vi "Empty_Complete.vi"(11 "input cluster":T1={"system"={"info"={"menuSelect"=0, "version"=0, "serial"="Test Sample", "captureActive"=FALSE, "captureBegin"=FALSE, "emptyAndRefill"=FALSE}, "userInfo"={"operatorName"="", "date"=timestamp(2713993200 s since 1904-01-01)}, "camera"={"exposureTime"=0, "aperture"=enum."Item 0", "framerate"=0, "framerateMax"=500, "legacyAttributes"=FALSE}}, "connections"={"arduino"={"connection"="MRJ", "status"=FALSE, "openState"=FALSE, "emptyStart"=0}, "pump"={"connection"="MRJ", "status"=FALSE, "command"="", "dispenseSpeed"=100, "flushSize"=100}, "camera"={"cam1"={"connection"="", "status"=FALSE}, "cam2"={"connection"="", "status"=FALSE}}}, "queue"={"process"={"cam1"=refnum, "cam2"=refnum, "queueSize"=0}, "save"={"cam1"=refnum, "cam2"=refnum, "queueSize"=0}, "overloadThreshold"=0}, "imageProcess"={"cam1"={"preAllocation"={"image"="Station", "originalDisplay"="Station", "originalRgb"="Station", "binary"="Station", "save"="Station", "calibrationFull"=refnum, "calibrationDetect"=refnum}, "calibration"={"pathFull"=path "C:/Users/au540322/Desktop/IHS_Project/images/Debris/Debris_0/Debris_0_2019_06_01-23-32-49-686.PNG", "pathDetect"=path "C:/Users/au540322/Desktop/IHS_Project/images/Debris/Debris_0/Debris_0_2019_06_01-23-32-49-686.PNG", "ROI"={"Left"=0, "Top"=0, "Right"=0, "Bottom"=0, "Rotation"=0.0}}}, "cam2"={"preAllocation"={"image"=refnum, "originalDisplay"=refnum, "originalRgb"=refnum, "binary"=refnum, "save"=refnum, "calibrationFull"=refnum, "calibrationDetect"=refnum}, "calibration"={"pathFull"=path "C:/Users/au540322/Desktop/IHS_Project/images/Debris/Debris_0/Debris_0_2019_06_01-23-32-49-686.PNG", "pathDetect"=path "C:/Users/au540322/Desktop/IHS_Project/images/Debris/Debris_0/Debris_0_2019_06_01-23-32-49-686.PNG", "ROI"={"Left"=0, "Top"=0, "Right"=0, "Bottom"=0, "Rotation"=0.0}}}, "process"={"planeExtract"=refnum, "planeSubtract"=refnum, "cropMask"=refnum}, "detection"={"sampleTimeout"=500, "sizeThreshold"=500, "detectionRegionPct"=0.0}}, "sampleData"={"sampleId"="", "projectId"="", "voucherID"="", "speciesName"="", "collectionDate"=timestamp(2713993200 s since 1904-01-01), "sampleStation"="", "location"="", "lat"=0.0, "lon"=0.0, "determiner"="", "sex"="", "otherNotes"=""}, "Session In"=""} {"sampleData"."collectionDate" format="%<%Y-%m-%d>T"; "imageProcess"."detection"."sizeThreshold" min=1; "imageProcess"."cam2"."calibration"."ROI"."Rotation" format="%.2f"; "imageProcess"."cam2"."calibration"."ROI"."Left" scale=0.0..1024.0; "imageProcess"."cam2"."calibration"."ROI"."Right" scale=0.0..1024.0; "imageProcess"."cam1"."calibration"."ROI"."Rotation" format="%.2f"; "imageProcess"."cam1"."calibration"."ROI"."Left" scale=0.0..1024.0; "imageProcess"."cam1"."calibration"."ROI"."Right" scale=0.0..1024.0; "queue"."overloadThreshold" min=1; "queue"."save"."queueSize" min=1; "queue"."process"."queueSize" min=1; "connections"."pump"."flushSize" min=1; "connections"."pump"."dispenseSpeed" min=1; "system"."camera"."framerateMax" min=1; "system"."userInfo"."date" format="%<%Y-%m-%dT%H:%M:%S+%z>T"; "system"."info"."version" items=["Standard", "XL"]; "system"."info"."menuSelect" items=["Session Data", "Extended Setup", "Buffer", "Camera", "Dispenser", "Stats", "Connections"]}) -> (0 "Next State":T5=enum."Pump Cycle", 3 "output cluster":T1={"system"={"info"={"menuSelect"=0, "version"=0, "serial"="Test Sample", "captureActive"=FALSE, "captureBegin"=FALSE, "emptyAndRefill"=FALSE}, "userInfo"={"operatorName"="", "date"=timestamp(2713993200 s since 1904-01-01)}, "camera"={"exposureTime"=0, "aperture"=enum."Item 0", "framerate"=0, "framerateMax"=500, "legacyAttributes"=FALSE}}, "connections"={"arduino"={"connection"="", "status"=FALSE, "openState"=FALSE, "emptyStart"=0}, "pump"={"connection"="", "status"=FALSE, "command"="", "dispenseSpeed"=100, "flushSize"=100}, "camera"={"cam1"={"connection"="", "status"=FALSE}, "cam2"={"connection"="", "status"=FALSE}}}, "queue"={"process"={"cam1"=refnum, "cam2"=refnum, "queueSize"=0}, "save"={"cam1"=refnum, "cam2"=refnum, "queueSize"=0}, "overloadThreshold"=0}, "imageProcess"={"cam1"={"preAllocation"={"image"="Station", "originalDisplay"="Station", "originalRgb"="Station", "binary"="Station", "save"="Station", "calibrationFull"=refnum, "calibrationDetect"=refnum}, "calibration"={"pathFull"=path "C:/Users/au540322/Desktop/IHS_Project/images/Debris/Debris_0/Debris_0_2019_06_01-23-32-49-686.PNG", "pathDetect"=path "C:/Users/au540322/Desktop/IHS_Project/images/Debris/Debris_0/Debris_0_2019_06_01-23-32-49-686.PNG", "ROI"={"Left"=0, "Top"=0, "Right"=0, "Bottom"=0, "Rotation"=0.0}}}, "cam2"={"preAllocation"={"image"=refnum, "originalDisplay"=refnum, "originalRgb"=refnum, "binary"=refnum, "save"=refnum, "calibrationFull"=refnum, "calibrationDetect"=refnum}, "calibration"={"pathFull"=path "C:/Users/au540322/Desktop/IHS_Project/images/Debris/Debris_0/Debris_0_2019_06_01-23-32-49-686.PNG", "pathDetect"=path "C:/Users/au540322/Desktop/IHS_Project/images/Debris/Debris_0/Debris_0_2019_06_01-23-32-49-686.PNG", "ROI"={"Left"=0, "Top"=0, "Right"=0, "Bottom"=0, "Rotation"=0.0}}}, "process"={"planeExtract"=refnum, "planeSubtract"=refnum, "cropMask"=refnum}, "detection"={"sampleTimeout"=500, "sizeThreshold"=500, "detectionRegionPct"=0.0}}, "sampleData"={"sampleId"="", "projectId"="", "voucherID"="", "speciesName"="", "collectionDate"=timestamp(2713993200 s since 1904-01-01), "sampleStation"="", "location"="", "lat"=0.0, "lon"=0.0, "determiner"="", "sex"="", "otherNotes"=""}, "Session In"=""} {"sampleData"."collectionDate" format="%<%Y-%m-%d>T"; "imageProcess"."detection"."sizeThreshold" min=1; "imageProcess"."cam2"."calibration"."ROI"."Rotation" format="%.2f"; "imageProcess"."cam2"."calibration"."ROI"."Left" scale=0.0..1024.0; "imageProcess"."cam2"."calibration"."ROI"."Right" scale=0.0..1024.0; "imageProcess"."cam1"."calibration"."ROI"."Rotation" format="%.2f"; "imageProcess"."cam1"."calibration"."ROI"."Left" scale=0.0..1024.0; "imageProcess"."cam1"."calibration"."ROI"."Right" scale=0.0..1024.0; "queue"."overloadThreshold" min=1; "queue"."save"."queueSize" min=1; "queue"."process"."queueSize" min=1; "connections"."pump"."flushSize" min=1; "connections"."pump"."dispenseSpeed" min=1; "system"."camera"."framerateMax" min=1; "system"."userInfo"."date" format="%<%Y-%m-%dT%H:%M:%S+%z>T"; "system"."info"."version" items=["Standard", "XL"]; "system"."info"."menuSelect" items=["Session Data", "Extended Setup", "Buffer", "Camera", "Dispenser", "Stats", "Connections"]})   [LabVIEW 2022 SP3]
uses:
  controls/Data.ctl
  <vilib>/userdefined/High Color/IMAQdx.ctl
  <vilib>/vision/Image Controls.llb/IMAQ Image.ctl
  controls/State.ctl
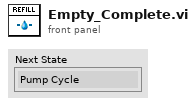
[diagram p1: front panel]
types:
  T1 = typedef "Data.ctl" = cluster{"system":cluster{"info":cluster{"menuSelect":u16, "version":u16, "serial":string, "captureActive":bool, "captureBegin":bool, "emptyAndRefill":bool}, "userInfo":cluster{"operatorName":string, "date":timestamp}, "camera":cluster{"exposureTime":i32, "aperture":enum32{"Item 0", "Item 1", "Item 2", "Item 3"}, "framerate":i32, "framerateMax":i32, "legacyAttributes":bool}}, "connections":cluster{"arduino":cluster{"connection":refnum<visa-resource-name>, "status":bool, "openState":bool, "emptyStart":u32}, "pump":cluster{"connection":refnum<visa-resource-name>, "status":bool, "command":string, "dispenseSpeed":i32, "flushSize":i32}, "camera":cluster{"cam1":cluster{"connection":T2, "status":bool}, "cam2":cluster{"connection":T2, "status":bool}}}, "queue":cluster{"process":cluster{"cam1":refnum<queue>, "cam2":refnum<queue>, "queueSize":i32}, "save":cluster{"cam1":refnum<queue>, "cam2":refnum<queue>, "queueSize":i32}, "overloadThreshold":i32}, "imageProcess":cluster{"cam1":cluster{"preAllocation":cluster{"image":T3, "originalDisplay":T3, "originalRgb":T3, "binary":T3, "save":T3, "calibrationFull":T3, "calibrationDetect":T3}, "calibration":cluster{"pathFull":path, "pathDetect":path, "ROI":T4}}, "cam2":cluster{"preAllocation":cluster{"image":T3, "originalDisplay":T3, "originalRgb":T3, "binary":T3, "save":T3, "calibrationFull":T3, "calibrationDetect":T3}, "calibration":cluster{"pathFull":path, "pathDetect":path, "ROI":T4}}, "process":cluster{"planeExtract":T3, "planeSubtract":T3, "cropMask":T3}, "detection":cluster{"sampleTimeout":i32, "sizeThreshold":i32, "detectionRegionPct":dbl}}, "sampleData":cluster{"sampleId":string, "projectId":string, "voucherID":string, "speciesName":string, "collectionDate":timestamp, "sampleStation":string, "location":string, "lat":dbl, "lon":dbl, "determiner":string, "sex":string, "otherNotes":string}, "Session In":T2}
  T2 = typedef "IMAQdx.ctl" = refnum<k21>
  T3 = typedef "IMAQ Image.ctl" = refnum<image>
  T4 = typedef "IMAQ Rectangle" = cluster{"Left":i32, "Top":i32, "Right":i32, "Bottom":i32, "Rotation":dbl}
  T5 = typedef "State.ctl" = enum16{"Initialize", "Wait for Event", "Position", "Valve Signal", "Extra Flush", "Valve Cycle", "Valve Open", "Valve Close", "Pump Command", "Pump Cycle", "Empty System", "Start System", "Connect Systems", "Start Image Capture", "Stop Image Capture", "Calibration Pictures", "Close and Refill", "Empty and Refill", "Change Light Intensity", "Reconnect", "CursorIdle", "Exit"}
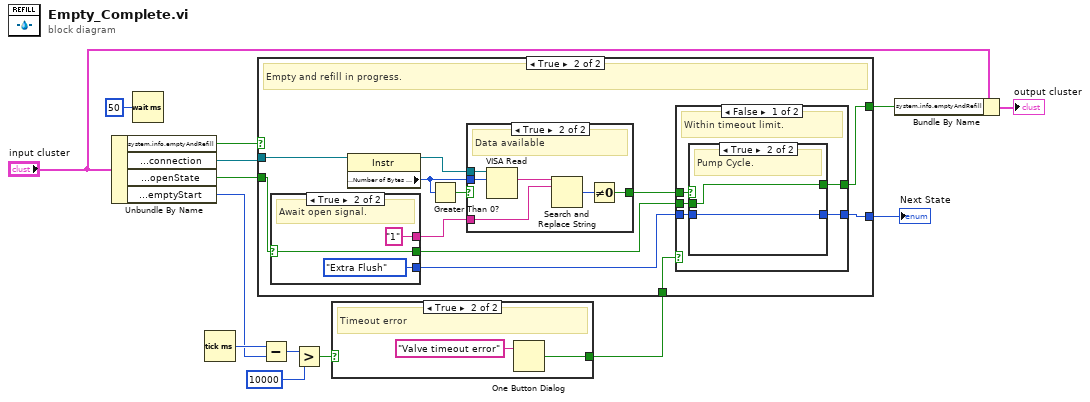
[diagram p0: block diagram]
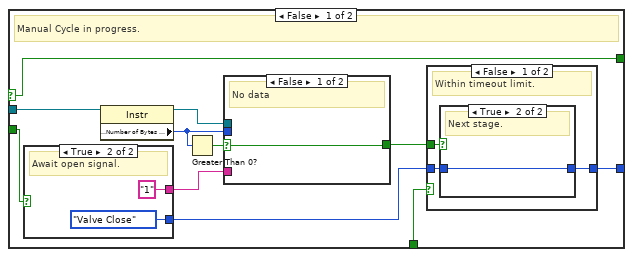
[diagram p3: hidden frame]
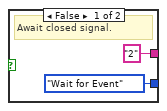
[diagram p4: hidden frame]
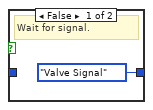
[diagram p5: hidden frame]
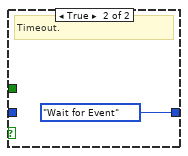
[diagram p6: hidden frame]
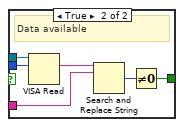
[diagram p7: hidden frame]
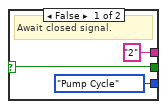
[diagram p8: hidden frame]
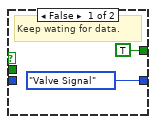
[diagram p9: hidden frame]
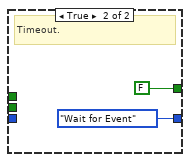
[diagram p10: hidden frame]
diagram:
  n1 = Unbundle By Name("input cluster") -> ("system.info.emptyAndRefill"=w14:bool, "connections.arduino.connection"=w13:refnum<visa-resource-name>, "connections.arduino.openState"=w1:bool, "connections.arduino.emptyStart"=w5:u32)
  n2 = Wait (ms)(milliseconds to wait=u32 50) -> ()  [unwired: 1 out]
  n3 = Tick Count (ms)() -> (millisecond timer value=w12:u32)
  n4 = Subtract(x=w12, y=w5) -> (x-y=w11:u32)
  n5 = Greater?(x=w11, y=u32 10000 ("x")) -> (0:w9:bool)
  n6 = case shown="True" w9 {
    selector: w9 -> [w15 _]
    tunnel: [w15 w16] -> w6
    frame False {
      # "Within timeout limit."
    }
    frame True {
      # "Timeout error"
      n7 = One Button Dialog(message="Valve timeout error") -> (true=w16:bool)  [unwired: 1 in]
    }
  }
  n8 = case shown="True" w14 {
    selector: w14 -> [w18 _]
    tunnel: w13 -> [w25 w54]
    tunnel: [w24 w53] -> w7
    tunnel: w6 -> [w23 w52]
    tunnel: [w18 w50] -> w3
    tunnel: w1 -> [w20 w49]
    frame False {
      # "Manual Cycle in progress."
      n9 = case shown="True" w20 {
        tunnel: ["2" ("y") "1" ("y")] -> w21
        tunnel: [State."Wait for Event" ("Next State") State."Valve Close" ("Next State")] -> w19
        frame False {
          # "Await closed signal."
        }
        frame True {
          # "Await open signal."
        }
      }
      n10 = property class="Instr"(reference=w25) -> (reference out=w26:refnum<visa-resource-name>, "Serial Settings:Number of Bytes at Serial Port"=w27:u32)  [unwired: 1 in, 1 out]
      n11 = Greater Than 0?(x=w27) -> (x > 0?=w28:bool)
      n12 = case shown="False" w28 {
        selector: w28 -> [w39 _]
        tunnel: w27 -> [_ w45]
        tunnel: w26 -> [_ w44]
        tunnel: [w39 w43] -> w22
        tunnel: w21 -> [_ w40]
        frame False {
          # "No data"
        }
        frame True {
          # "Data available"
          n13 = VISA Read(VISA resource name=w44, byte count=w45) -> (read buffer=w42:string)  [unwired: 1 in, 3 out]
          n14 = Search and Replace String(input string=w42, search string=w40) -> (number of replacements=w41:i32)  [unwired: 6 in, 3 out]
          n15 = Not Equal To 0?(x=w41) -> (x != 0?=w43:bool)
        }
      }
      n16 = case shown="False" w23 {
        tunnel: [w35 State."Wait for Event" ("Next State")] -> w24
        tunnel: w22 -> [w34 _]
        tunnel: w19 -> [w33 _]
        frame False {
          # "Within timeout limit."
          n17 = case shown="True" w34 {
            tunnel: [State."Valve Signal" ("Next State") w37] -> w35
            tunnel: w33 -> [_ w37]
            frame False {
              # "Wait for signal."
            }
            frame True {
              # "Next stage."
            }
          }
        }
        frame True {
          # "Timeout."
        }
      }
    }
    frame True {
      # "Empty and refill in progress."
      n18 = case shown="True" w49 {
        selector: w49 -> [w58 w61]
        tunnel: ["2" ("y") "1" ("y")] -> w48
        tunnel: [State."Pump Cycle" ("Next State") State."Extra Flush" ("Next State")] -> w47
        tunnel: [w58 w61] -> w46
        frame False {
          # "Await closed signal."
        }
        frame True {
          # "Await open signal."
        }
      }
      n19 = property class="Instr"(reference=w54) -> (reference out=w55:refnum<visa-resource-name>, "Serial Settings:Number of Bytes at Serial Port"=w56:u32)  [unwired: 1 in, 1 out]
      n20 = Greater Than 0?(x=w56) -> (x > 0?=w57:bool)
      n21 = case shown="True" w57 {
        selector: w57 -> [w75 _]
        tunnel: w56 -> [_ w81]
        tunnel: w55 -> [_ w80]
        tunnel: [w75 w79] -> w51
        tunnel: w48 -> [_ w76]
        frame False {
          # "No data"
        }
        frame True {
          # "Data available"
          n22 = VISA Read(VISA resource name=w80, byte count=w81) -> (read buffer=w78:string)  [unwired: 1 in, 3 out]
          n23 = Search and Replace String(input string=w78, search string=w76) -> (number of replacements=w77:i32)  [unwired: 6 in, 3 out]
          n24 = Not Equal To 0?(x=w77) -> (x != 0?=w79:bool)
        }
      }
      n25 = case shown="False" w52 {
        tunnel: [w68 State."Wait for Event" ("Next State")] -> w53
        tunnel: w51 -> [w67 _]
        tunnel: [w66 FALSE] -> w50
        tunnel: w47 -> [w65 _]
        tunnel: w46 -> [w64 _]
        frame False {
          # "Within timeout limit."
          n26 = case shown="True" w67 {
            tunnel: [State."Valve Signal" ("Next State") w72] -> w68
            tunnel: [TRUE w71] -> w66
            tunnel: w65 -> [_ w72]
            tunnel: w64 -> [_ w71]
            frame False {
              # "Keep wating for data."
            }
            frame True {
              # "Pump Cycle."
            }
          }
        }
        frame True {
          # "Timeout."
        }
      }
    }
  }
  "Next State" <- w7
  n27 = Bundle By Name(cluster="input cluster", "system.info.emptyAndRefill"=w3) -> (→"output cluster":T1)
